vi "Angle_2.vi"() -> ()   [LabVIEW 2020]
uses:
  Support/Controls/Cmd_Mouse Popup.ctl
  Support/Controls/Clst_Initialize Input.ctl
  Support/Controls/Clst_Result inspec.ctl
  Support/Controls/Cmd_Var Data IO.ctl
  Variables/Global_Cal Info.vi
panel:
  out "Meas 2_calcu":string[][](table) caption="좌측 눈금 계산값"
  out "Meas 1_calcu":string[][](table) caption="우측 눈금 계산값"
  in  "부기포관 위치":string(combo)
  out "눈금수":string
  out "Resolution 2":string[][](table) caption="Resolution"
  out "Spec 2":string[][](table) caption="Spec"
  out "Condition 2":string[][](table) caption="● 기준선의 좌측 눈금"
  in  "Measured 2":string[][](table) caption="수준기 눈금 읽음값"
  out "단위":string
  out "최대범위":string
  in  "Spec 변경":bool
  in  "Random":bool
  out "Resolution":string[][](table)
  out "Spec":string[][](table)
  out "제목":string
  out "에러 출력":errorcluster
  out "Condition":string[][](table) caption="● 기준선의 우측 눈금"
  in  "최소눈금":string(combo)
  in  "Measured":string[][](table) caption="수준기 눈금 읽음값"
  out "Load?":bool
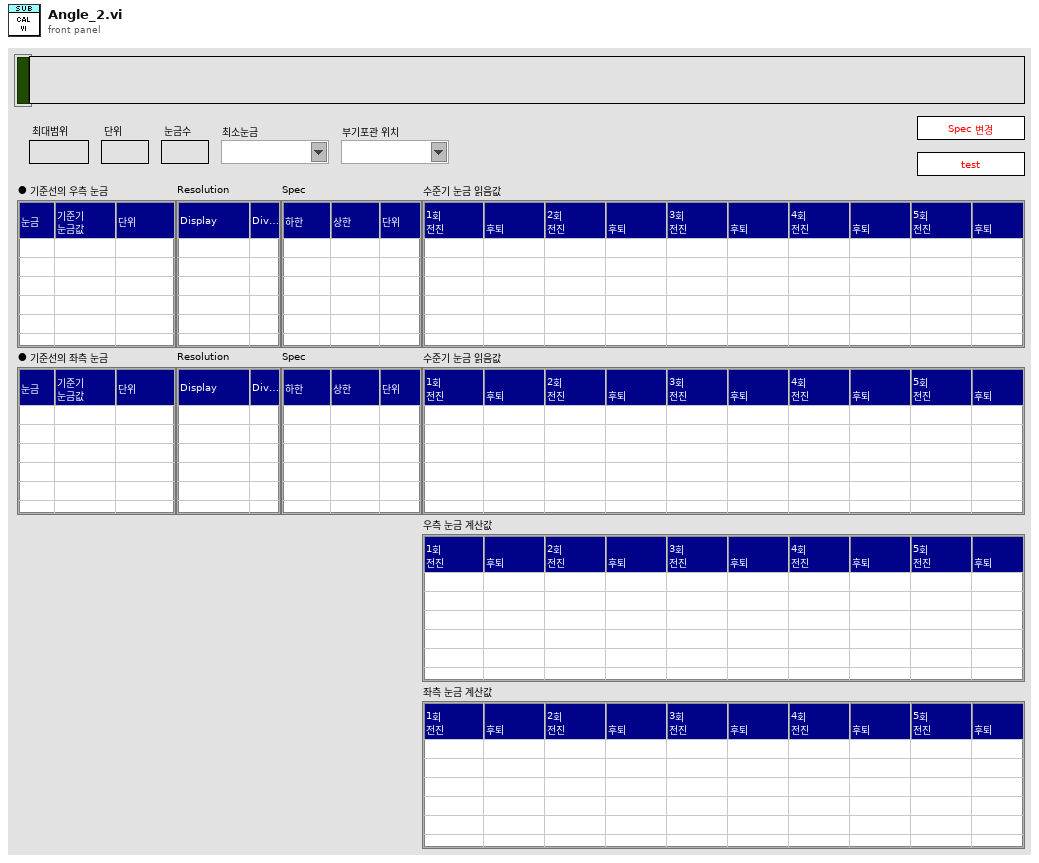
[diagram p1: front panel]
types:
  T1 = typedef "Cmd_Mouse Popup.ctl" = enum16{"활성화", "메뉴선택"}
  T2 = cluster{"Shift":bool, "Ctrl":bool, "Alt":bool, "Cmd":bool, "Opt":bool}
  T3 = typedef "Clst_Initialize Input.ctl" = cluster{"Initialize 1":cluster{"Condition":refnum<vi>[], "Spec":refnum<vi>[], "Measured":refnum<vi>[], "Resolution":refnum<vi>[], "Func_ext":string, "제목":refnum<vi>, "Measured_ADJ":refnum<vi>[]}, "Initialize 2":cluster{"문자열":refnum<vi>[], "콤보박스":refnum<vi>[], "링":refnum<vi>[], "열거형":refnum<vi>[], "테이블":refnum<vi>[], "여러열":refnum<vi>[], "디지털(DBL)":refnum<vi>[], "3D string":refnum<vi>[], "ctrl":refnum<vi>[], "boolean":refnum<vi>[]}}
  T4 = typedef "Clst_Result inspec.ctl" = cluster{"분해능":string, "문자열 1":string, "문자열 2":string, "숫자형 1":i32, "숫자형 2":i32, "숫자형 3":dbl, "문자배열 1D":string[], "문자배열 2D":string[][], "문자배열 3D":string[][][], "문자배열 4D":string[][][][], "불리언 1D":bool[]}
  T5 = typedef "Cmd_Var Data IO.ctl" = enum16{"Condition", "Condition Default", "Condition_Temp", "Resolution", "Resolution Default", "Resolution Old", "Spec", "Spec Default", "Spec Old", "Spec Temp", "Result", "Result2", "Result3", "Result_Temp", "Result_ADJ", "Result_ADJ2", "STD1", "STD2", "STD3", "STD4", "STD5", "STD Temp", "CMC", "CMC Default"}
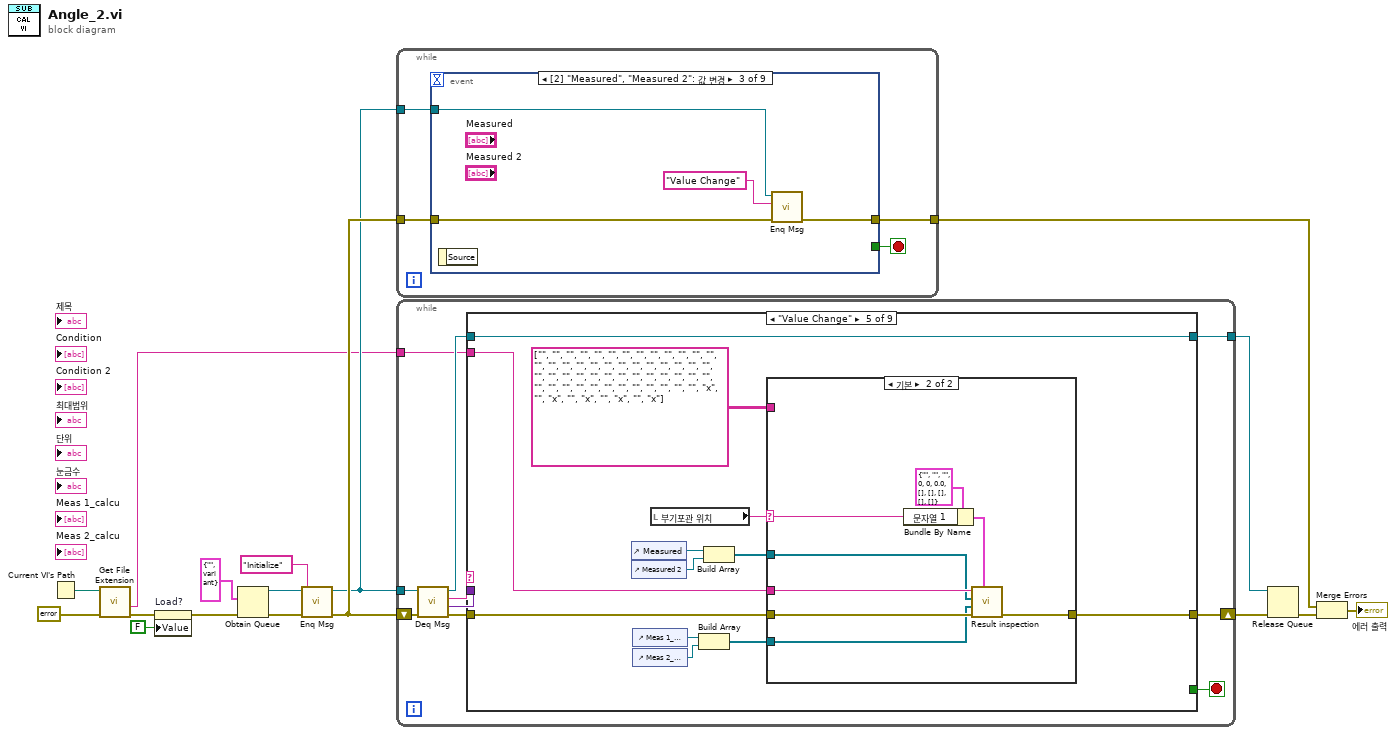
[diagram p0: block diagram]
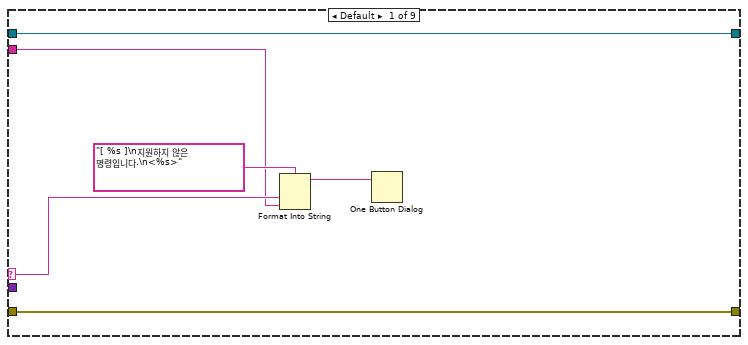
[diagram p2: hidden frame]
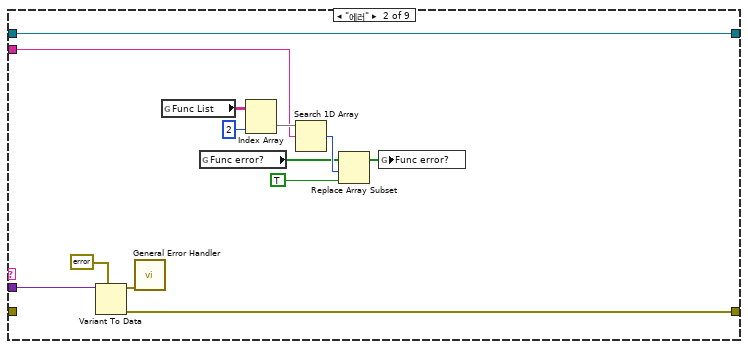
[diagram p3: hidden frame]
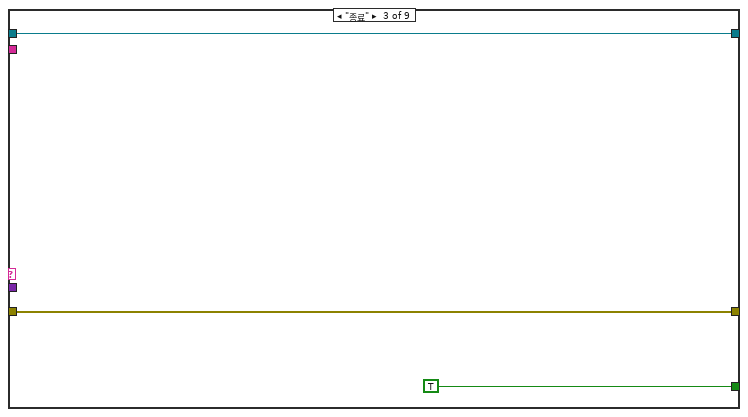
[diagram p4: hidden frame]
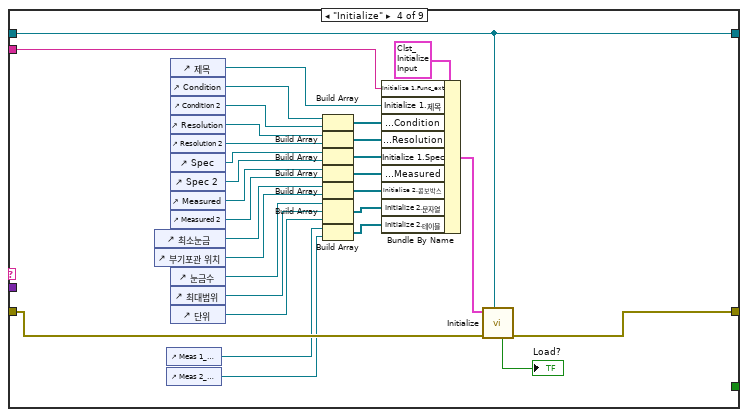
[diagram p5: hidden frame]
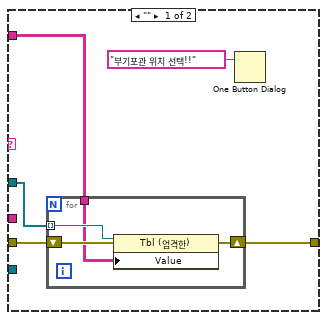
[diagram p6: hidden frame]
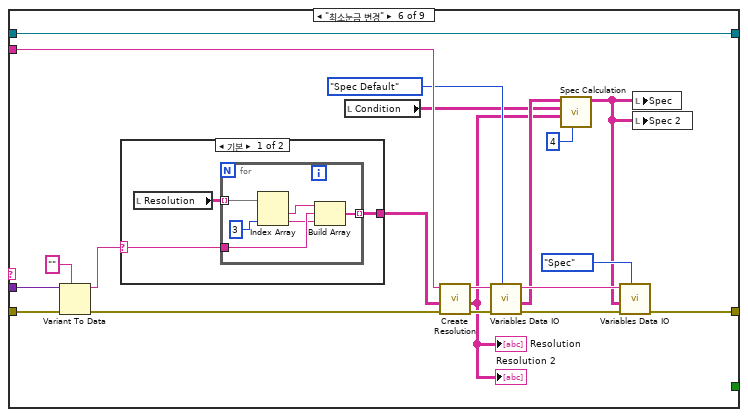
[diagram p7: hidden frame]
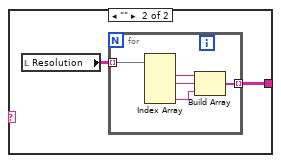
[diagram p8: hidden frame]
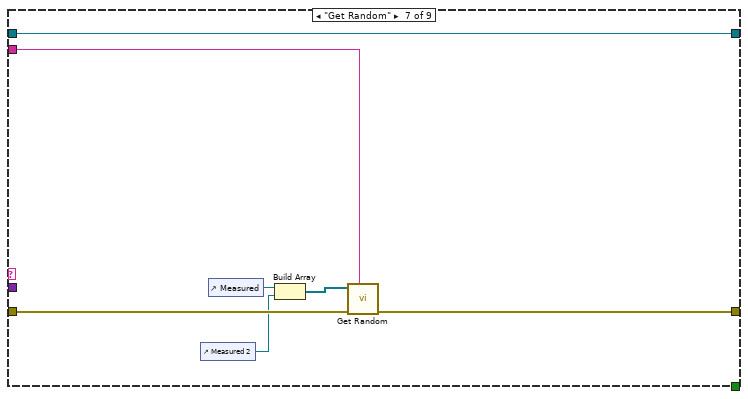
[diagram p9: hidden frame]
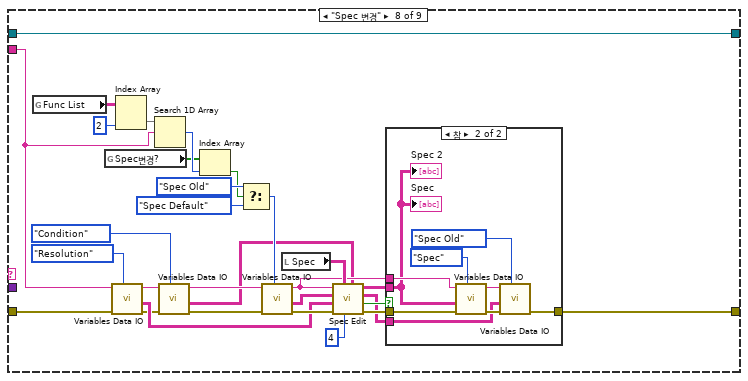
[diagram p10: hidden frame]
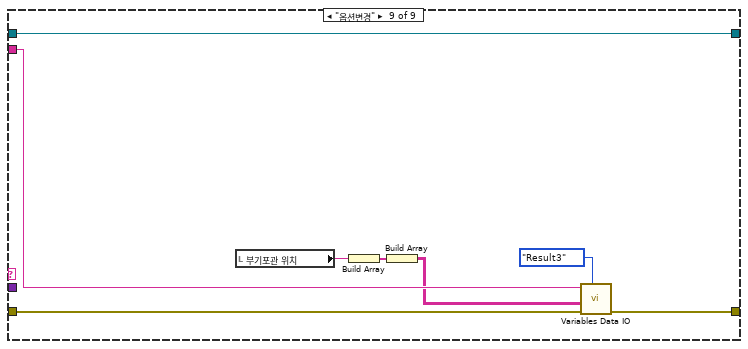
[diagram p12: hidden frame]
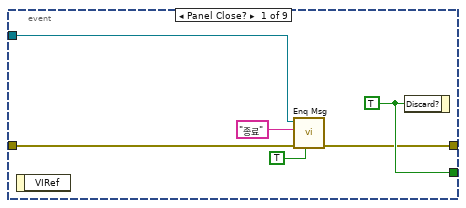
[diagram p13: hidden frame]
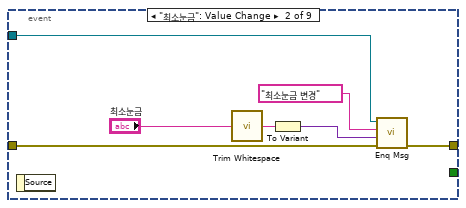
[diagram p14: hidden frame]
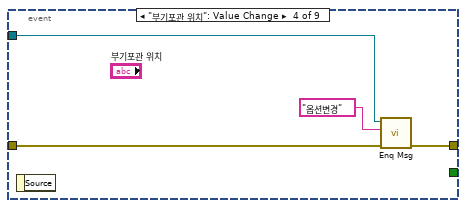
[diagram p15: hidden frame]
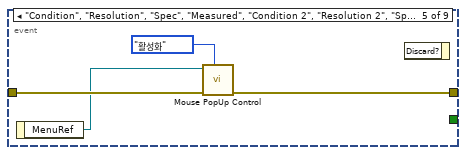
[diagram p16: hidden frame]
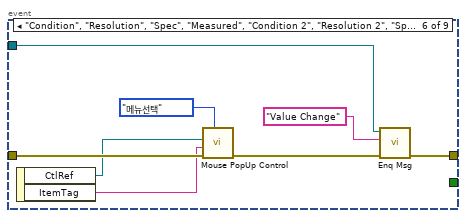
[diagram p17: hidden frame]
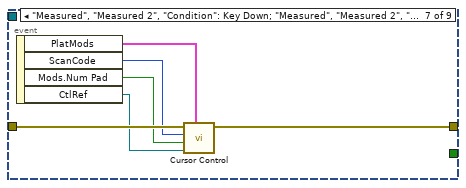
[diagram p18: hidden frame]
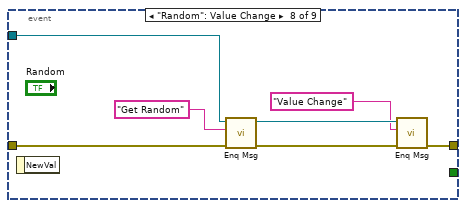
[diagram p19: hidden frame]
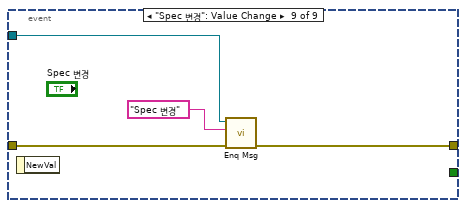
[diagram p20: hidden frame]
diagram:
  n1 = Current VI's Path() -> (path=w5:path)
  n2 = call <vilib>:"Get File Extension.vi"("error in (no error)"=errorcluster {"status"=FALSE, "code"=0, "source"=""} ("에러 상수"), "file"=w5) -> ("error out"=w3:errorcluster, "filename without extension"=w4:string)  [unwired: 5 in, 3 out]
  n3 = property on="Load?" class="Bool (엄격한)"(error in=w3, "Value"=FALSE ("Load?")) -> (error out=w2:errorcluster)  [unwired: 1 in, 1 out]
  n4 = Obtain Queue(element data type=cluster{"메세지":string, "값":variant} {"메세지"="", "값"=variant} ("Message Cluster"), error in (no error)=w2) -> (queue out=w14:refnum<queue>, error out=w16:errorcluster)  [unwired: 3 in, 1 out]
  n5 = call "Enq Msg.vi"("에러 입력(에러 없음)"=w16, "메세지"="Initialize", "큐 입력"=w14) -> ("에러 출력"=w15:errorcluster, "큐 출력"=w12:refnum<queue>)  [unwired: 7 in]
  n6 = while {
    tunnel: w15 -> [w19]
    tunnel: w12 -> [w20]
    tunnel: [w18] -> w9
    stop <- w21 stop-if-true
    n7 = event shown="[2] \"Measured\", \"Measured 2\": 값 변경" {
      selector: _ -> [_ _ _ _ _ _ _ _ _]
      dyn-events: _ -> [_ _ _ _ _ _ _ _ _]
      timeout: _ -> [_ _ _ _ _ _ _ _ _]
      tunnel: [w27 _ _ _ _ _ _ _ _] -> w21
      tunnel: w20 -> [w25 w33 w38 w39 _ w47 _ w65 w69]
      tunnel: w19 -> [w26 w34 w36 w41 w46 w54 w60 w66 w70]
      tunnel: [w23 w32 w37 w40 w45 w48 w59 w61 w68] -> w18
      event Panel Close? {
        w27 = TRUE ("버림?")
        n8 = event-data() -> ()  [unwired: 1 in, 1 out]
        n9 = call "Enq Msg.vi"("우선순위 메시지?"=TRUE, "에러 입력(에러 없음)"=w26, "메세지"="종료", "큐 입력"=w25) -> ("에러 출력"=w23:errorcluster)  [unwired: 6 in, 1 out]
        n10 = event-data("Discard?"=w27) -> ()  [unwired: 1 in, 1 out]
      }
      event "최소눈금": Value Change {
        n11 = event-data() -> ()  [unwired: 1 in, 1 out]
        n12 = call <vilib>:"Trim Whitespace.vi"("string"="최소눈금") -> ("trimmed string"=w30:string)  [unwired: 1 in]
        n13 = To Variant(anything=w30) -> (Variant=w28:variant)
        n14 = call "Enq Msg.vi"("에러 입력(에러 없음)"=w34, "값"=w28, "메세지"="최소눈금 변경", "큐 입력"=w33) -> ("에러 출력"=w32:errorcluster)  [unwired: 6 in, 1 out]
      }
      event "Measured", "Measured 2": Value Change {
        n15 = event-data() -> ()  [unwired: 1 in, 1 out]
        n16 = call "Enq Msg.vi"("에러 입력(에러 없음)"=w36, "메세지"="Value Change", "큐 입력"=w38) -> ("에러 출력"=w37:errorcluster)  [unwired: 7 in, 1 out]
      }
      event "부기포관 위치": Value Change {
        n17 = event-data() -> ()  [unwired: 1 in, 1 out]
        n18 = call "Enq Msg.vi"("에러 입력(에러 없음)"=w41, "메세지"="옵션변경", "큐 입력"=w39) -> ("에러 출력"=w40:errorcluster)  [unwired: 7 in, 1 out]
      }
      event "Condition", "Resolution", "Spec", "Measured", "Condition 2", "Resolution 2", "Spec 2", "Measured 2": Shortcut Menu Activation? {
        n19 = event-data() -> ("MenuRef"=w44:refnum<k9>)  [unwired: 1 in]
        n20 = call "Mouse PopUp Control.vi"("type"=Cmd_Mouse_Popup."활성화", "error in"=w46, "메뉴 참조"=w44) -> ("error out"=w45:errorcluster)  [unwired: 8 in]
        n21 = event-data() -> ()  [unwired: 2 in, 1 out]
      }
      event "Condition", "Resolution", "Spec", "Measured", "Condition 2", "Resolution 2", "Spec 2", "Measured 2": Shortcut Menu Selection (User) {
        n22 = event-data() -> ("CtlRef"=w52:refnum<vi>, "ItemTag"=w51:string)  [unwired: 1 in]
        n23 = call "Mouse PopUp Control.vi"("type"=Cmd_Mouse_Popup."메뉴선택", "error in"=w54, "아이템 태그"=w51, "Tbl 참조 번호"=w52) -> ("error out"=w49:errorcluster)  [unwired: 7 in]
        n24 = call "Enq Msg.vi"("에러 입력(에러 없음)"=w49, "메세지"="Value Change", "큐 입력"=w47) -> ("에러 출력"=w48:errorcluster)  [unwired: 7 in, 1 out]
      }
      event "Measured", "Measured 2", "Condition": Key Down; "Measured", "Measured 2", "Condition": Key Repeat {
        n25 = event-data() -> ("PlatMods"=w55:T2, "ScanCode"=w58:i16, "Mods.Num Pad"=w57:bool, "CtlRef"=w56:refnum<vi>)  [unwired: 1 in]
        n26 = call "Cursor Control.vi"("플랫폼 조합키"=w55, "참조"=w56, "Num Pad"=w57, "ScanCode"=w58, "error in"=w60) -> ("error out"=w59:errorcluster)  [unwired: 5 in, 1 out]
      }
      event "Random": Value Change {
        n27 = event-data() -> ()  [unwired: 1 in, 1 out]
        n28 = call "Enq Msg.vi"("에러 입력(에러 없음)"=w66, "메세지"="Get Random", "큐 입력"=w65) -> ("에러 출력"=w64:errorcluster, "큐 출력"=w63:refnum<queue>)  [unwired: 7 in]
        n29 = call "Enq Msg.vi"("에러 입력(에러 없음)"=w64, "메세지"="Value Change", "큐 입력"=w63) -> ("에러 출력"=w61:errorcluster)  [unwired: 7 in, 1 out]
      }
      event "Spec 변경": Value Change {
        n30 = event-data() -> ()  [unwired: 1 in, 1 out]
        n31 = call "Enq Msg.vi"("에러 입력(에러 없음)"=w70, "메세지"="Spec 변경", "큐 입력"=w69) -> ("에러 출력"=w68:errorcluster)  [unwired: 7 in, 1 out]
      }
    }
  }
  n32 = while {
    shift-right: [w81] -> w11
    shift-left: w15 -> [w80]
    tunnel: w12 -> [w78]
    tunnel: [w73] -> w10
    tunnel: w4 -> [w72]
    stop <- w74 stop-if-true
    n33 = call "Deq Msg.vi"("에러 입력(에러 없음)"=w80, "큐 입력"=w78) -> ("에러 출력"=w79:errorcluster, "값"=w75:variant, "메세지"=w77:string, "큐 출력"=w76:refnum<queue>)  [unwired: 6 in]
    n34 = case shown="\"Value Change\"" w77 {
      selector: w77 -> [w83 _ _ _ _ _ _ _ _]
      tunnel: w79 -> [w87 _ w103 w133 w142 w181 w201 w228 w252]
      tunnel: [w87 w97 w103 w124 w144 w175 w202 w231 w251] -> w81
      tunnel: w76 -> [w86 w96 w101 w118 w145 w182 w205 w235 w253]
      tunnel: w75 -> [_ w98 _ _ _ w180 _ _ _]
      tunnel: [_ _ TRUE ("버림?") _ _ _ _ _ _] -> w74
      tunnel: [w86 w96 w101 w118 w145 w182 w205 w235 w253] -> w73
      tunnel: w72 -> [w82 w88 _ w119 w143 w178 w200 w213 w250]
      frame Default {
        n35 = Format Into String(format string="[ %s ]\n지원하지 않은 명령입니다.\n<%s>" ("메시지"), w83, w82) -> (resulting string=w84:string)  [unwired: 2 in, 1 out]
        n36 = One Button Dialog(message=w84) -> ()  [unwired: 1 in, 1 out]
      }
      frame "에러" {
        n37 = Variant To Data(type=errorcluster {"status"=FALSE, "code"=0, "source"=""} ("에러 출력"), Variant=w98) -> (data=w100:errorcluster, error out=w97:errorcluster)  [unwired: 1 in]
        n38 = call <vilib>:"General Error Handler.vi"("error in (no error)"=w100) -> ()  [unwired: 10 in, 5 out]
        n39 = global read "Global_Cal Info.vi" "Func List"() -> (w90:string[][])
        n40 = global read "Global_Cal Info.vi" "Func error?"() -> (w93:bool[])
        n41 = Index Array(array=w90, index (col)=2 ("비활성화된 인덱스 (열)")) -> (element=w91:string[])  [unwired: 1 in]
        n42 = Search 1D Array(1D array=w91, element=w88) -> (index of element=w94:i32)  [unwired: 1 in]
        n43 = Replace Array Subset(array=w93, new element=TRUE ("새 원소/부분배열"), index=w94) -> (w95:bool[])
        n44 = global write "Global_Cal Info.vi" "Func error?"(w95) -> ()
      }
      frame "종료" {
      }
      frame "Initialize" {
        n45 = control-ref of="최소눈금"() -> (w117:refnum<vi>)
        n46 = control-ref of="부기포관 위치"() -> (w108:refnum<vi>)
        n47 = control-ref of="Meas 1_calcu"() -> (w106:refnum<vi>)
        n48 = control-ref of="Meas 2_calcu"() -> (w105:refnum<vi>)
        n49 = control-ref of="제목"() -> (w125:refnum<vi>)
        n50 = control-ref of="Condition"() -> (w130:refnum<vi>)
        n51 = control-ref of="Condition 2"() -> (w113:refnum<vi>)
        n52 = control-ref of="Resolution"() -> (w120:refnum<vi>)
        n53 = control-ref of="Resolution 2"() -> (w112:refnum<vi>)
        n54 = control-ref of="Spec"() -> (w123:refnum<vi>)
        n55 = control-ref of="Spec 2"() -> (w111:refnum<vi>)
        n56 = control-ref of="Measured"() -> (w127:refnum<vi>)
        n57 = control-ref of="Measured 2"() -> (w110:refnum<vi>)
        n58 = control-ref of="눈금수"() -> (w109:refnum<vi>)
        n59 = control-ref of="최대범위"() -> (w114:refnum<vi>)
        n60 = control-ref of="단위"() -> (w116:refnum<vi>)
        n61 = Build Array(w130, w113) -> (w129:refnum<vi>[])
        n62 = Build Array(w120, w112) -> (w121:refnum<vi>[])
        n63 = Build Array(w123, w111) -> (w122:refnum<vi>[])
        n64 = Build Array(w127, w110) -> (w128:refnum<vi>[])
        n65 = Build Array(w117, w108) -> (w126:refnum<vi>[])
        n66 = Build Array(w109, w114, w116) -> (w115:refnum<vi>[])
        n67 = Build Array(w106, w105) -> (w104:refnum<vi>[])
        n68 = Bundle By Name(cluster=T3 {"Initialize 1"={"Condition"=[], "Spec"=[], "Measured"=[], "Resolution"=[], "Func_ext"="", "제목"=refnum, "Measured_ADJ"=[]}, "Initialize 2"={"문자열"=[], "콤보박스"=[], "링"=[], "열거형"=[], "테이블"=[], "여러열"=[], "디지털(DBL)"=[], "3D string"=[], "ctrl"=[], "boolean"=[]}} ("입력 클러스터"), "Initialize 1.Func_ext"=w119, "Initialize 1.제목"=w125, "Initialize 1.Condition"=w129, "Initialize 1.Resolution"=w121, "Initialize 1.Spec"=w122, "Initialize 1.Measured"=w128, "Initialize 2.콤보박스"=w126, "Initialize 2.문자열"=w115, "Initialize 2.테이블"=w104) -> (w131:T3)
        n69 = call "Initialize.vi"("큐 입력"=w118, "error in"=w133, "입력 클러스터"=w131) -> ("error out"=w124:errorcluster, "Load?"=→"Load?":bool)  [unwired: 5 in, 2 out]
      }
      frame "Value Change" {
        n70 = control-ref of="Measured"() -> (w139:refnum<vi>)
        n71 = control-ref of="Measured 2"() -> (w140:refnum<vi>)
        n72 = control-ref of="Meas 1_calcu"() -> (w137:refnum<vi>)
        n73 = control-ref of="Meas 2_calcu"() -> (w136:refnum<vi>)
        n74 = local read "부기포관 위치"() -> (w141:string)
        n75 = Build Array(w137, w136) -> (w135:refnum<vi>[])
        n76 = Build Array(w139, w140) -> (w138:refnum<vi>[])
        n77 = case shown="기본" w141 {
          selector: w141 -> [_ w156]
          tunnel: [w148 w162] -> w144
          tunnel: w143 -> [_ w161]
          tunnel: w142 -> [w150 w160]
          tunnel: w138 -> [w149 w159]
          tunnel: w135 -> [_ w158]
          tunnel: string[][] [["", "", "", "", "", "", "", "", "", ""], ["", "", "", "", "", "", "", "", "", ""], ["", "", "", "", "", "", "", "", "", ""], ["", "", "", "", "", "", "", "", "", ""], ["", "", "", "", "", "", "", "", "", ""], ["", "ⅹ", "", "ⅹ", "", "ⅹ", "", "ⅹ", "", "ⅹ"]] ("Measured") -> [w147 _]
          frame "" {
            n78 = for {
              tunnel: w149 -> [w153] mode=indexing
              shift-right: [w152] -> w148
              shift-left: w150 -> [w154]
              tunnel: w147 -> [w151]
              n79 = property class="Tbl (엄격한)"(reference=w153, error in=w154, "Value"=w151) -> (error out=w152:errorcluster)  [unwired: 1 out]
            }
            n80 = One Button Dialog(message="부기포관 위치 선택!!" ("메시지")) -> ()  [unwired: 1 in, 1 out]
          }
          frame Default {
            n81 = Bundle By Name(cluster=T4 {"분해능"="", "문자열 1"="", "문자열 2"="", "숫자형 1"=0, "숫자형 2"=0, "숫자형 3"=0.0, "문자배열 1D"=[], "문자배열 2D"=[], "문자배열 3D"=[], "문자배열 4D"=[], "불리언 1D"=[]} ("입력 클러스터"), "문자열 1"=w156) -> (w155:T4)
            n82 = call "Result inspection.vi"("입력 클러스터"=w155, "error in"=w160, "Ref. Data (excluded)"=w158, "Ref. Data (Inspection)"=w159, "Func ext"=w161) -> ("error out"=w162:errorcluster)  [unwired: 3 in, 3 out]
          }
        }
      }
      frame "최소눈금 변경" {
        n83 = Variant To Data(error in=w181, type="", Variant=w180) -> (data=w165:string, error out=w168:errorcluster)
        n84 = case shown="기본" w165 {
          selector: w165 -> [w183 _]
          tunnel: [w185 w193] -> w167
          frame Default {
            n85 = local read "Resolution"() -> (w184:string[][])
            n86 = for {
              tunnel: w184 -> [w191] mode=indexing
              tunnel: w183 -> [w190]
              tunnel: [w188] -> w185 mode=indexing
              n87 = Index Array(array=w191, index #2=3 ("인덱스")) -> (element #1=w186:string, element #2=w189:string)  [unwired: 1 in]
              n88 = Build Array(w186, w190, w189) -> (w188:string[])
            }
          }
          frame "" {
            n89 = local read "Resolution"() -> (w192:string[][])
            n90 = for {
              tunnel: w192 -> [w198] mode=indexing
              tunnel: [w197] -> w193 mode=indexing
              n91 = Index Array(array=w198) -> (element #1=w194:string, element #2=w196:string, element #4=w195:string)  [unwired: 4 in, 1 out]
              n92 = Build Array(w194, w196, w195) -> (w197:string[])
            }
          }
        }
        n93 = local read "Condition"() -> (w166:string[][])
        n94 = call "Create Resolution.vi"("에러 입력(에러 없음)"=w168, "Resolution"=w167, "Func_ext"=w178) -> ("에러 출력"=w173:errorcluster, "Resolution Out"=w164:string[][], "Func_ext 출력"=w171:string)  [unwired: 6 in]
        "Resolution" <- w164
        "Resolution 2" <- w164
        n95 = call "Variables Data IO.vi"("Select"=Cmd_Var_Data_IO."Spec Default", "error in"=w173, "Func_ext"=w171) -> ("error out"=w172:errorcluster, "Data Out"=w169:string[][], "Func_ext Out"=w170:string)  [unwired: 6 in]
        n96 = call "Spec Calculation.vi"("기준값 열번호"=4 ("열번호(기준값)"), "Resolution"=w164, "Condition in"=w166, "Spec Default"=w169) -> ("Spec out"=w163:string[][])  [unwired: 6 in, 1 out]
        n97 = call "Variables Data IO.vi"("Select"=Cmd_Var_Data_IO."Spec", "error in"=w172, "Data In"=w163, "Func_ext"=w170) -> ("error out"=w175:errorcluster)  [unwired: 5 in, 2 out]
        n98 = local write "Spec"(w163) -> ()
        n99 = local write "Spec 2"(w163) -> ()
      }
      frame "Get Random" {
        n100 = control-ref of="Measured 2"() -> (w199:refnum<vi>)
        n101 = control-ref of="Measured"() -> (w204:refnum<vi>)
        n102 = Build Array(w204, w199) -> (w203:refnum<vi>[])
        n103 = call "Get Random.vi"("Func_Ext"=w200, "에러 입력"=w201, "Meas"=w203) -> ("에러 출력"=w202:errorcluster)  [unwired: 7 in, 1 out]
      }
      frame "Spec 변경" {
        n104 = global read "Global_Cal Info.vi" "Func List"() -> (w218:string[][])
        n105 = global read "Global_Cal Info.vi" "Spec변경?"() -> (w214:bool[])
        n106 = call "Variables Data IO.vi"("Select"=Cmd_Var_Data_IO."Resolution", "error in"=w228, "Func_ext"=w213) -> ("error out"=w211:errorcluster, "Data Out"=w222:string[][], "Func_ext Out"=w209:string)  [unwired: 6 in]
        n107 = Index Array(array=w218, index (col)=2 ("비활성화된 인덱스 (열)")) -> (element=w216:string[])  [unwired: 1 in]
        n108 = Search 1D Array(1D array=w216, element=w213) -> (index of element=w215:i32)  [unwired: 1 in]
        n109 = call "Variables Data IO.vi"("Select"=Cmd_Var_Data_IO."Condition", "error in"=w211, "Func_ext"=w209) -> ("error out"=w210:errorcluster, "Data Out"=w206:string[][], "Func_ext Out"=w208:string)  [unwired: 6 in]
        n110 = Index Array(array=w214, index=w215) -> (element=w219:bool)
        n111 = Select(t=Cmd_Var_Data_IO."Spec Old" ("Select"), s=w219, f=Cmd_Var_Data_IO."Spec Default" ("Select")) -> (s? t:f=w212:T5)
        n112 = call "Variables Data IO.vi"("Select"=w212, "error in"=w210, "Func_ext"=w208) -> ("error out"=w230:errorcluster, "Data Out"=w223:string[][], "Func_ext Out"=w224:string)  [unwired: 6 in]
        n113 = local read "Spec"() -> (w225:string[][])
        n114 = call "Spec Edit.vi"("Condition"=w206, "열번호(기준값)"=4, "Spec Value"=w225, "에러 입력(에러 없음)"=w230, "Resolution"=w222, "Spec Default"=w223, "Func_ext"=w224) -> ("에러 출력"=w232:errorcluster, "변경?"=w233:bool, "Spec Default out"=w227:string[][], "Spec 출력"=w234:string[][])  [unwired: 1 in]
        n115 = case shown="참" w233 {
          tunnel: w234 -> [_ w237]
          tunnel: w232 -> [w236 w245]
          tunnel: [w236 w241] -> w231
          tunnel: w224 -> [_ w243]
          tunnel: w227 -> [_ w239]
          frame False {
          }
          frame True {
            n116 = call "Variables Data IO.vi"("Select"=Cmd_Var_Data_IO."Spec", "error in"=w245, "Data In"=w237, "Func_ext"=w243) -> ("error out"=w242:errorcluster, "Func_ext Out"=w240:string)  [unwired: 5 in, 1 out]
            n117 = call "Variables Data IO.vi"("Select"=Cmd_Var_Data_IO."Spec Old", "error in"=w242, "Data In"=w239, "Func_ext"=w240) -> ("error out"=w241:errorcluster)  [unwired: 5 in, 2 out]
            "Spec" <- w237
            "Spec 2" <- w237
          }
        }
      }
      frame "옵션변경" {
        n118 = local read "부기포관 위치"() -> (w248:string)
        n119 = Build Array(w248) -> (w247:string[])
        n120 = Build Array(w247) -> (w246:string[][])
        n121 = call "Variables Data IO.vi"("Select"=Cmd_Var_Data_IO."Result3", "error in"=w252, "Data In"=w246, "Func_ext"=w250) -> ("error out"=w251:errorcluster)  [unwired: 5 in, 2 out]
      }
    }
  }
  n122 = Release Queue(queue=w10, error in (no error)=w11) -> (error out=w8:errorcluster)  [unwired: 1 in, 2 out]
  n123 = Merge Errors(w9, w8) -> (→"에러 출력":errorcluster)
